vi "GestureSensor PAJ7620U2.vi"() -> ()   [LabVIEW 2024]
uses:
  Driver/Public/Digital Pull Direction.ctl
  51c12f6e-4a21-4d98-9fb3-1a2e6b8270e3.vi
  d8ff4ad1-6435-4902-b67c-6ac0edf8525d.vi
  Driver/CTIPicoVISA.lvlib
panel:
  out "Pict Ring":u16(ring)
  out "loop":i32
  out "43":u8 format="%08b"
  out "Identity":T1
  out "Init Data":string
  in  "Grove Connector":enum16{"I2C0", "I2C1"}(ring)
  in  "stop":bool
  in  "VISA resource name in":refnum<visa-resource-name>="COM7"
  out "error out":errorcluster
  # "https://www.seeedstudio.com/Grove-Gesture-PAJ7620U2.html"
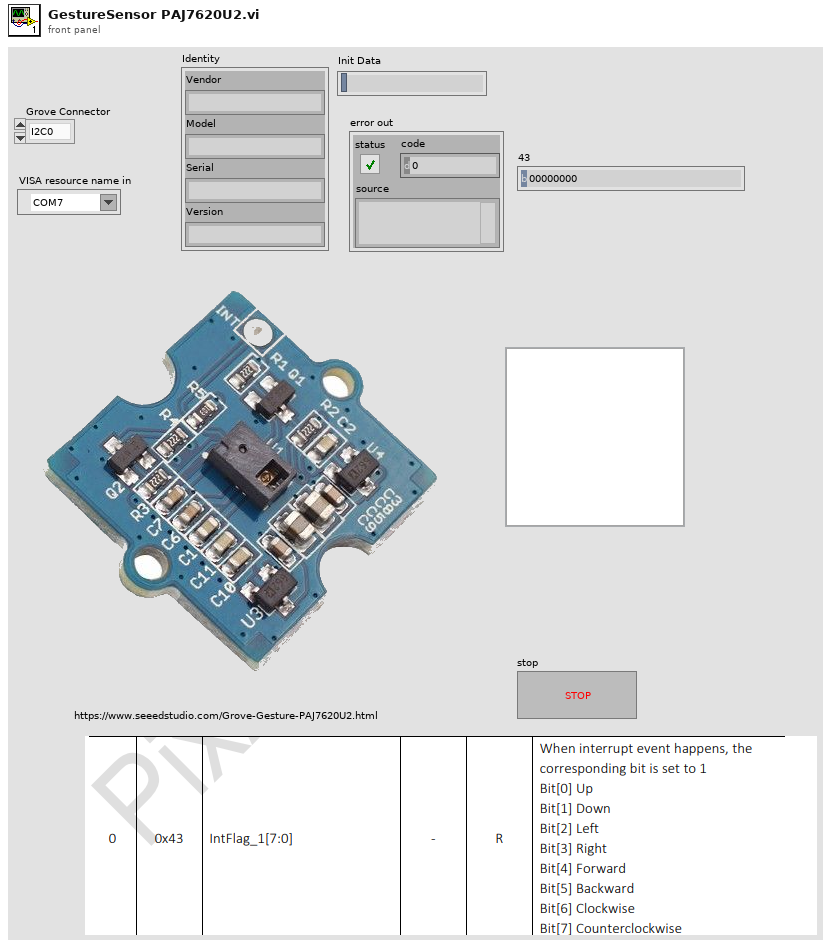
[diagram p1: front panel]
types:
  T1 = cluster{"Vendor":string, "Model":string, "Serial":string, "Version":string}
  T2 = typedef "CTIPicoVISA.lvlib/Digital Pull Direction.ctl" = enum16{"None", "Up", "Down", "Both"}
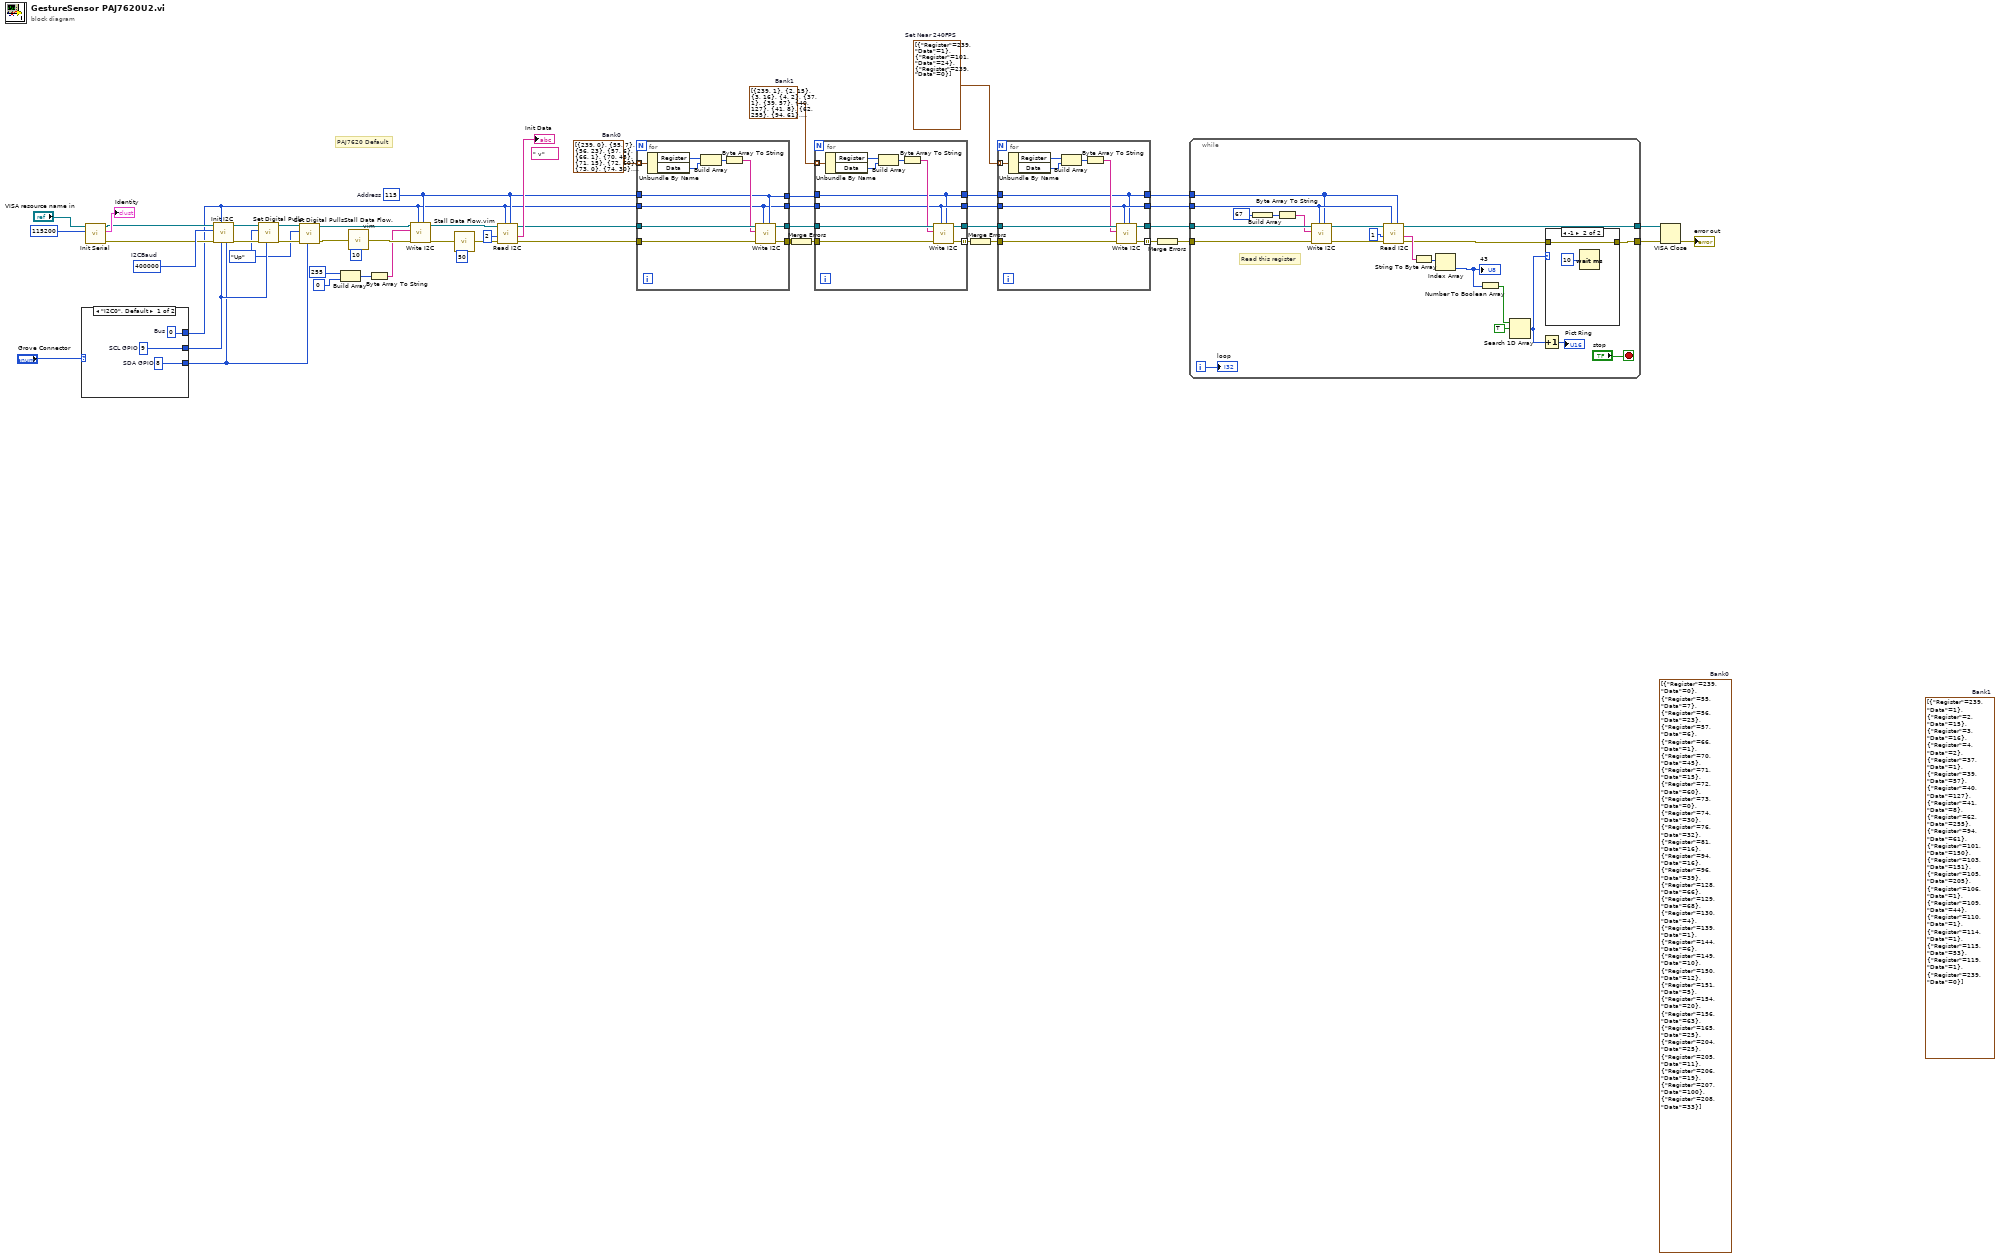
[diagram p0: block diagram]
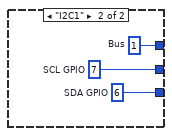
[diagram p2: hidden frame]
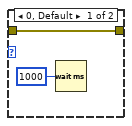
[diagram p3: hidden frame]
diagram:
  (unwired) cluster{"Register":u8, "Data":u8}[] [{"Register"=239, "Data"=0}, {"Register"=55, "Data"=7}, {"Register"=56, "Data"=23}, {"Register"=57, "Data"=6}, {"Register"=66, "Data"=1}, {"Register"=70, "Data"=45}, {"Register"=71, "Data"=15}, {"Register"=72, "Data"=60}, {"Register"=73, "Data"=0}, {"Register"=74, "Data"=30}, {"Register"=76, "Data"=32}, {"Register"=81, "Data"=16}, {"Register"=94, "Data"=16}, {"Register"=96, "Data"=39}, {"Register"=128, "Data"=66}, {"Register"=129, "Data"=68}, {"Register"=130, "Data"=4}, {"Register"=139, "Data"=1}, {"Register"=144, "Data"=6}, {"Register"=149, "Data"=10}, {"Register"=150, "Data"=12}, {"Register"=151, "Data"=5}, {"Register"=154, "Data"=20}, {"Register"=156, "Data"=63}, {"Register"=165, "Data"=25}, {"Register"=204, "Data"=25}, {"Register"=205, "Data"=11}, {"Register"=206, "Data"=19}, {"Register"=207, "Data"=100}, {"Register"=208, "Data"=33}]  # Bank0
  (unwired) cluster{"Register":u8, "Data":u8}[] [{"Register"=239, "Data"=1}, {"Register"=2, "Data"=15}, {"Register"=3, "Data"=16}, {"Register"=4, "Data"=2}, {"Register"=37, "Data"=1}, {"Register"=39, "Data"=57}, {"Register"=40, "Data"=127}, {"Register"=41, "Data"=8}, {"Register"=62, "Data"=255}, {"Register"=94, "Data"=61}, {"Register"=101, "Data"=150}, {"Register"=103, "Data"=151}, {"Register"=105, "Data"=205}, {"Register"=106, "Data"=1}, {"Register"=109, "Data"=44}, {"Register"=110, "Data"=1}, {"Register"=114, "Data"=1}, {"Register"=115, "Data"=53}, {"Register"=119, "Data"=1}, {"Register"=239, "Data"=0}]  # Bank1
  w8 = cluster{"Register":u8, "Data":u8}[] [{"Register"=239, "Data"=1}, {"Register"=101, "Data"=24}, {"Register"=239, "Data"=0}]  # Set Near 240FPS
  w18 = cluster{"Register":u8, "Data":u8}[] [{"Register"=239, "Data"=1}, {"Register"=2, "Data"=15}, {"Register"=3, "Data"=16}, {"Register"=4, "Data"=2}, {"Register"=37, "Data"=1}, {"Register"=39, "Data"=57}, {"Register"=40, "Data"=127}, {"Register"=41, "Data"=8}, {"Register"=62, "Data"=255}, {"Register"=94, "Data"=61}, {"Register"=101, "Data"=150}, {"Register"=103, "Data"=151}, {"Register"=105, "Data"=205}, {"Register"=106, "Data"=1}, {"Register"=109, "Data"=44}, {"Register"=110, "Data"=1}, {"Register"=114, "Data"=1}, {"Register"=115, "Data"=53}, {"Register"=119, "Data"=1}, {"Register"=239, "Data"=0}]  # Bank1
  w25 = cluster{"Register":u8, "Data":u8}[] [{"Register"=239, "Data"=0}, {"Register"=55, "Data"=7}, {"Register"=56, "Data"=23}, {"Register"=57, "Data"=6}, {"Register"=66, "Data"=1}, {"Register"=70, "Data"=45}, {"Register"=71, "Data"=15}, {"Register"=72, "Data"=60}, {"Register"=73, "Data"=0}, {"Register"=74, "Data"=30}, {"Register"=76, "Data"=32}, {"Register"=81, "Data"=16}, {"Register"=94, "Data"=16}, {"Register"=96, "Data"=39}, {"Register"=128, "Data"=66}, {"Register"=129, "Data"=68}, {"Register"=130, "Data"=4}, {"Register"=139, "Data"=1}, {"Register"=144, "Data"=6}, {"Register"=149, "Data"=10}, {"Register"=150, "Data"=12}, {"Register"=151, "Data"=5}, {"Register"=154, "Data"=20}, {"Register"=156, "Data"=63}, {"Register"=165, "Data"=25}, {"Register"=204, "Data"=25}, {"Register"=205, "Data"=11}, {"Register"=206, "Data"=19}, {"Register"=207, "Data"=100}, {"Register"=208, "Data"=33}]  # Bank0
  (unwired) " v" ("Init Data")
  w29 = Digital_Pull_Direction."Up" ("Pull")
  w22 = u8 115  # Address
  w50 = u32 400000  # I2CBaud
  # "PAJ7620 Default"
  n1 = case shown="\"I2C0\", Default" "Grove Connector" {
    tunnel: [w56 w59] -> w30
    tunnel: [w55 w58] -> w28
    tunnel: [w54 w57] -> w1
    frame "I2C0", Default {
      w54 = u8 0  # Bus
      w55 = 8  # SDA GPIO
      w56 = 9  # SCL GPIO
    }
    frame "I2C1" {
      w57 = u8 1  # Bus
      w58 = 6  # SDA GPIO
      w59 = 7  # SCL GPIO
    }
  }
  n2 = call "Init Serial.vi"("Baud (115200)"=u32 115200, "VISA resource name in"="VISA resource name in") -> ("error out"=w12:errorcluster, "Identity"=→"Identity":T1, "VISA resource name Out"=w13:refnum<visa-resource-name>)  [unwired: 7 in]
  n3 = call "Init I2C.vi"("SDA GPIO"=w28, "SCL GPIO"=w30, "Bus"=w1, "error in (no error)"=w12, "Baud"=w50, "VISA resource name in"=w13) -> ("error out"=w33:errorcluster, "VISA resource name"=w34:refnum<visa-resource-name>)  [unwired: 4 in]
  n4 = call "Set Digital Pulls.vi"("GPIO"=w30, "error in (no error)"=w33, "Pull"=w29, "VISA resource name in"=w34) -> ("error out"=w31:errorcluster, "VISA resource name"=w32:refnum<visa-resource-name>)  [unwired: 6 in]
  n5 = call "Set Digital Pulls.vi"("GPIO"=w28, "error in (no error)"=w31, "Pull"=w29, "VISA resource name in"=w32) -> ("error out"=w26:errorcluster, "VISA resource name"=w27:refnum<visa-resource-name>)  [unwired: 6 in]
  n6 = Build Array(u8 255 ("Value"), u8 0 ("Value")) -> (w47:u8[])
  n7 = call "Stall Data Flow.vim"("value in"=w26, "milliseconds to wait"=u32 10) -> ("value out"=w44:errorcluster)  [unwired: 1 out]
  n8 = Byte Array To String(unsigned byte array=w47) -> (string=w43:string)
  n9 = call "Write I2C.vi"("Address"=w22, "Bus"=w1, "error in (no error)"=w44, "Data"=w43, "VISA resource name in"=w27) -> ("error out"=w41:errorcluster, "VISA resource name"=w40:refnum<visa-resource-name>)  [unwired: 5 in]
  n10 = call "Stall Data Flow.vim"("value in"=w41, "milliseconds to wait"=u32 50) -> ("value out"=w39:errorcluster)  [unwired: 1 out]
  n11 = call "Read I2C.vi"("Address"=w22, "Bus"=w1, "error in (no error)"=w39, "Len"=u8 2, "VISA resource name in"=w40) -> ("error out"=w24:errorcluster, "Data"=→"Init Data":string, "VISA resource name"=w23:refnum<visa-resource-name>)  [unwired: 4 in]
  n12 = for {
    tunnel: w25 -> [w67] mode=indexing
    tunnel: w24 -> [w69]
    tunnel: w23 -> [w70]
    tunnel: w1 -> [w60]
    tunnel: w22 -> [w61]
    tunnel: [w63] -> w21
    tunnel: [w62] -> _ mode=indexing
    tunnel: [w62] -> w20
    tunnel: [w61] -> w16
    tunnel: [w60] -> w15
    n13 = Unbundle By Name(w67) -> ("Register"=w66:u8, "Data"=w65:u8)
    n14 = Build Array(w66, w65) -> (w68:u8[])
    n15 = Byte Array To String(unsigned byte array=w68) -> (string=w64:string)
    n16 = call "Write I2C.vi"("Address"=w61, "Bus"=w60, "error in (no error)"=w69, "Data"=w64, "VISA resource name in"=w70) -> ("error out"=w62:errorcluster, "VISA resource name"=w63:refnum<visa-resource-name>)  [unwired: 5 in]
  }
  n17 = Merge Errors(w20) -> (w19:errorcluster)
  n18 = for {
    tunnel: w18 -> [w78] mode=indexing
    tunnel: w19 -> [w80]
    tunnel: w21 -> [w81]
    tunnel: w15 -> [w72]
    tunnel: w16 -> [w71]
    tunnel: [w74] -> w10
    tunnel: [w73] -> w17 mode=indexing
    tunnel: [w72] -> w9
    tunnel: [w71] -> w7
    n19 = Unbundle By Name(w78) -> ("Register"=w77:u8, "Data"=w76:u8)
    n20 = Build Array(w77, w76) -> (w79:u8[])
    n21 = Byte Array To String(unsigned byte array=w79) -> (string=w75:string)
    n22 = call "Write I2C.vi"("Address"=w71, "Bus"=w72, "error in (no error)"=w80, "Data"=w75, "VISA resource name in"=w81) -> ("error out"=w73:errorcluster, "VISA resource name"=w74:refnum<visa-resource-name>)  [unwired: 5 in]
  }
  n23 = Merge Errors(w17) -> (w11:errorcluster)
  n24 = for {
    tunnel: w8 -> [w89] mode=indexing
    tunnel: w11 -> [w91]
    tunnel: w10 -> [w92]
    tunnel: w9 -> [w83]
    tunnel: w7 -> [w82]
    tunnel: [w85] -> w4
    tunnel: [w84] -> w6 mode=indexing
    tunnel: [w83] -> w3
    tunnel: [w82] -> w2
    n25 = Unbundle By Name(w89) -> ("Register"=w88:u8, "Data"=w87:u8)
    n26 = Build Array(w88, w87) -> (w90:u8[])
    n27 = Byte Array To String(unsigned byte array=w90) -> (string=w86:string)
    n28 = call "Write I2C.vi"("Address"=w82, "Bus"=w83, "error in (no error)"=w91, "Data"=w86, "VISA resource name in"=w92) -> ("error out"=w84:errorcluster, "VISA resource name"=w85:refnum<visa-resource-name>)  [unwired: 5 in]
  }
  n29 = Merge Errors(w6) -> (w5:errorcluster)
  n30 = while {
    tunnel: w5 -> [w108]
    tunnel: [w95] -> w36
    tunnel: w4 -> [w109]
    tunnel: [w113] -> w35
    tunnel: w3 -> [w105]
    tunnel: w2 -> [w104]
    i -> [w100]
    stop <- "stop" stop-if-true
    # "Read this register"
    n31 = Build Array(u8 67 ("Register")) -> (w103:u8[])
    n32 = Byte Array To String(unsigned byte array=w103) -> (string=w101:string)
    n33 = call "Write I2C.vi"("Address"=w104, "Bus"=w105, "error in (no error)"=w108, "Data"=w101, "VISA resource name in"=w109) -> ("error out"=w107:errorcluster, "VISA resource name"=w106:refnum<visa-resource-name>)  [unwired: 5 in]
    n34 = call "Read I2C.vi"("Address"=w104, "Bus"=w105, "error in (no error)"=w107, "Len"=u8 1, "VISA resource name in"=w106) -> ("error out"=w96:errorcluster, "Data"=w112:string, "VISA resource name"=w113:refnum<visa-resource-name>)  [unwired: 4 in]
    n35 = String To Byte Array(string=w112) -> (unsigned byte array=w111:u8[])
    n36 = Index Array(array=w111) -> (element=w110:u8)  [unwired: 1 in]
    "43" <- w110
    n37 = Number To Boolean Array(number=w110) -> (Boolean array=w98:bool[])
    n38 = Search 1D Array(1D array=w98, element=TRUE) -> (index of element=w93:i32)  [unwired: 1 in]
    n39 = Increment(x=w93) -> (x+1=→"Pict Ring":i32)
    n40 = case shown="-1" w93 {
      tunnel: w96 -> [w115 w118]
      tunnel: [w115 w118] -> w95
      frame 0, Default {
        n41 = Wait (ms)(milliseconds to wait=u32 1000) -> ()  [unwired: 1 out]
      }
      frame -1 {
        n42 = Wait (ms)(milliseconds to wait=u32 10) -> ()  [unwired: 1 out]
      }
    }
    "loop" <- w100
  }
  n43 = VISA Close(VISA resource name=w35, error in (no error)=w36) -> (error out=→"error out":errorcluster)
